vi "offset.get.vi"(8 "error in (no error)":errorcluster, 11 "ts.relative in":refnum<class "ts.relative.lvclass">) -> (0 "error out":errorcluster, 2 "offset":timestamp format="%<%x %.3X>T", 3 "ts.relative out":refnum<class "ts.relative.lvclass">)   [LabVIEW 2020, in "ts.relative.lvclass"]
uses:
  ts.relative.lvclass
  ts.relative.lvclass/ts.relative.ctl
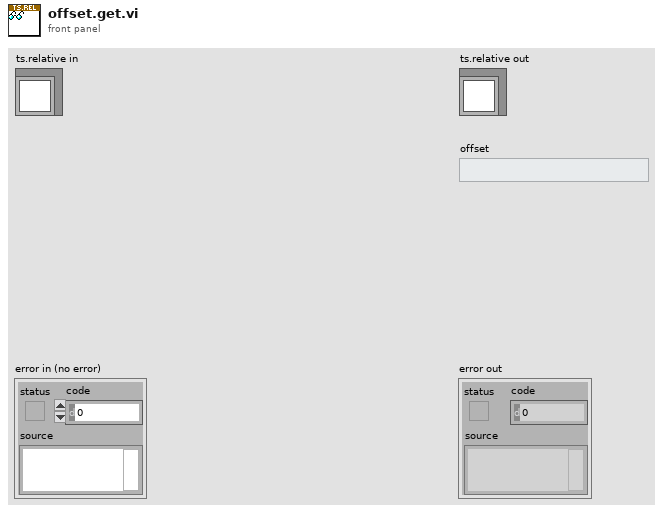
[diagram p1: front panel]
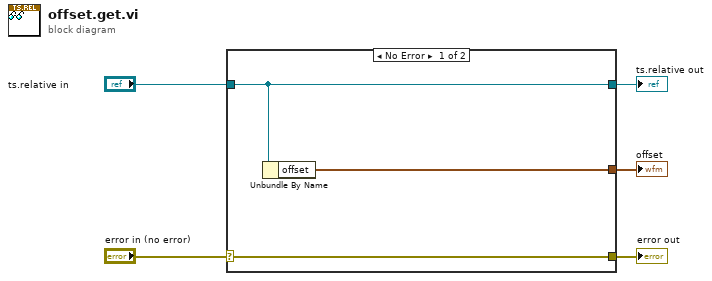
[diagram p0: block diagram]
diagram:
  n1 = case shown="No Error" "error in (no error)" {
    selector: "error in (no error)" -> [w8 w9]
    tunnel: [w8 w9] -> w4
    tunnel: [w7 w10] -> w2
    tunnel: "ts.relative in" -> [w7 w10]
    tunnel: [w6 _] -> w1
    frame No Error {
      n2 = Unbundle By Name(w7) -> ("offset"=w6:timestamp)
    }
    frame Error {
    }
  }
  "error out" <- w4
  "ts.relative out" <- w2
  "offset" <- w1
